vi "observacao_0MQ.vi"() -> ()   [LabVIEW 2012, in "Shared_160.lvlib"] (continued)
              tunnel: w81 -> [_ w133]
              frame False {
              }
              frame True {
                w134 = "\t"
                # "CÚPULA TRAVADA: Write LOG"
                n304 = String To Path(string="C:\\TCS\\LOG\\CUPULA\\TRAVOU.TXT" ("pathLogFocoString")) -> (path=w142:path)
                n305 = Open/Create/Replace File(file path (use dialog)=w142, error in=errorcluster {"status"=FALSE, "code"=0, "source"=""}, operation (0:open)=T7."open or create") -> (refnum out=w129:refnum<file>, error out=w127:errorcluster)  [unwired: 3 in, 1 out]
                n306 = Get Date/Time String(date format (0)=enum16{"short", "long", "abbreviated"}."short", want seconds? (F)=TRUE) -> (date string=w136:string, time string=w135:string)  [unwired: 1 in]
                n307 = Build Array(w136, w134, w135, w134, "ETIQUETA: ", w133, "\r\n") -> (w130:string[])
                n308 = call "TickTimeout.vi"() -> ("msTick"=w122:u32)  [unwired: 2 in, 2 out]
                n309 = Set File Position(refnum=w129, from (0:start)=enum16{"start", "end", "current"}."end", error in=w127) -> (refnum out=w128:refnum<file>, error out=w126:errorcluster)  [unwired: 1 in]
                n310 = global write "Global_Telescopio.vi" "CupTimeLock"(w122) -> ()
                n311 = Write to Text File(file (use dialog)=w128, text=w130, error in=w126) -> (refnum out=w139:refnum<file>, error out=w140:errorcluster)  [unwired: 1 in, 1 out]
                n312 = Close File(refnum=w139, error in=w140) -> ()  [unwired: 2 out]
              }
            }
            n313 = Or(x=w93, y=w94) -> (x .or. y?=w92:bool)
            n314 = Tick Count (ms)() -> (millisecond timer value=w87:u32)
            n315 = Add(x=w89, y=40000) -> (x+y=w86:i32)
            n316 = Greater Or Equal?(x=w87, y=w86) -> (x >= y?=w85:bool)
            n317 = shared-variable "My Computer\\Shared_160.lvlib\\Beep"(w92) -> ()  [unwired: 1 in, 1 out]
            n318 = And(x=w85, y=w84) -> (x .and. y?=w83:bool)
            n319 = case shown="True" w83 {
              frame False {
              }
              frame True {
                w203 = u16 4 items=["ZERO", "AH", "DEC", "TUBO", "CUP"] ("Controlador")
                # "Envia o comando para o\ncontrolador da cupula, após 40 segundos"
                n320 = local write "sendCommandShutter"(FALSE ("writeShutterLog")) -> ()
                n321 = call "Monta Comando.vi"("Comando"="PARAR", "Dispositivo"="TRAPEIRA" ("Comando"), "Controlador"=w203) -> ()  [unwired: 4 in, 3 out]
              }
            }
            n322 = call "Sideral_Time.vi"("Fuso"=-3.0) -> ("TU"=→"UT":string, "Sideral Time"=w110:dbl)  [unwired: 2 in, 1 out]
            n323 = global write "Global_Telescopio.vi" "Sideral Time"(w110) -> ()
          }
          frame #1 {
            w317 = u16 9 items=["Alarme", "Atencao", "Erro", "Ocupado", "Protecao", "Embreagem", "Tracking", "Var. Track", "Rápido", "Ligeiro", "Médio", "Lento", "Em movimento", ""] ("NomeStatus")
            w318 = u16 9 items=["Alarme", "Atencao", "Erro", "Ocupado", "Protecao", "Embreagem", "Tracking", "Var. Track", "Rápido", "Ligeiro", "Médio", "Lento", "Em movimento", ""] ("NomeStatus")
            w321 = u16 8 items=["Alarme", "Atencao", "Erro", "Ocupado", "Protecao", "Embreagem", "Tracking", "Var. Track", "Rápido", "Ligeiro", "Médio", "Lento", "Em movimento", ""] ("NomeStatus")
            w322 = u16 8 items=["Alarme", "Atencao", "Erro", "Ocupado", "Protecao", "Embreagem", "Tracking", "Var. Track", "Rápido", "Ligeiro", "Médio", "Lento", "Em movimento", ""] ("NomeStatus")
            w328 = 6.283185307179586
            # "Desabilita botões \"Precess\" e \"Clear\"\ndurante o apontamento"
            # "MUDANÇA:\nBit EMBREAGEM trocado pelos bits RAPIDO e LIGEIRO para detectar a retirada do objeto da posição centrada."
            # "MUDANÇA FUTURA:\nTrocar globais de calagem por valores \"latch\" dessas globais. Finalidade: manter display de coordenadas consistentes mesmo quando o usuário zerar as calagens, especialmente a local, para o próximo apontamento."
            # "ATUALIZA \nINDICADORES \nDO PAINEL"
            n324 = local read "ChkCalGlobal"() -> (w333:bool)
            n325 = global read "Global_Telescopio.vi" "PosDEC"() -> (w336:dbl)
            n326 = global read "Global_Telescopio.vi" "Sideral Time"() -> (w338:dbl)
            n327 = global read "Global_Telescopio.vi" "ObjCentrado"() -> (w310:bool)
            "ObjCentrado" <- w310
            n328 = global read "Global_Telescopio.vi" "PosAH"() -> (w337:dbl)
            n329 = call "Calcula epoch.vi"() -> ("epoch"=→"Epoch":dbl)  [unwired: 2 in]
            n330 = call "Bit Status AH.vi"("NomeStatus"=w322) -> ("StatBit"=w320:bool)
            n331 = call "Bit Status AH.vi"("NomeStatus"=w317) -> ("StatBit"=w316:bool)
            n332 = call "Bit Status DEC.vi"("NomeStatus"=w321) -> ("StatBit"=w314:bool)
            n333 = call "Bit Status DEC.vi"("NomeStatus"=w318) -> ("StatBit"=w315:bool)
            n334 = local read "LedPointing"() -> (w305:bool)
            n335 = Tick Count (ms)() -> (millisecond timer value=w306:u32)
            n336 = Compound Arithmetic op=OR(w320, w316, w314, w315) -> (w319:bool)
            n337 = case shown="True" w319 {
              frame False {
              }
              frame True {
                n338 = global write "Global_Telescopio.vi" "ObjCentrado"(FALSE) -> ()
              }
            }
            n339 = case shown="False" w305 {
              frame False {
                w344 = 0
                n340 = property on="BtPointPrecess" class="Bool"("DisabledEnum"=w344) -> ()  [unwired: 2 in, 2 out]
                n341 = property on="BtPointObjClear" class="Bool"("DisabledEnum"=w344) -> ()  [unwired: 2 in, 2 out]
              }
              frame True {
                w345 = 2
                n342 = property on="BtPointPrecess" class="Bool"("DisabledEnum"=w345) -> ()  [unwired: 2 in, 2 out]
                n343 = property on="BtPointObjClear" class="Bool"("DisabledEnum"=w345) -> ()  [unwired: 2 in, 2 out]
              }
            }
            n344 = case shown="True" w310 {
              tunnel: [w415 w432] -> w330
              tunnel: [w414 w431] -> w326
              tunnel: [w417 w435] -> w304
              tunnel: [w416 w433] -> w323
              tunnel: w338 -> [w415 w432]
              tunnel: w337 -> [w420 _]
              tunnel: w336 -> [w419 _]
              tunnel: w333 -> [w418 _]
              tunnel: [w413 w429] -> _
              tunnel: w306 -> [w413 w429]
              frame False {
                n345 = case shown="True" w418 {
                  tunnel: w419 -> [w422 w428]
                  tunnel: [w422 w427] -> w417
                  tunnel: w420 -> [w421 w426]
                  tunnel: [w421 w423] -> w416
                  frame False {
                  }
                  frame True {
                    n346 = global read "Global_Telescopio.vi" "Calagem AH"() -> (w424:dbl)
                    n347 = global read "Global_Telescopio.vi" "Calagem DEC"() -> (w425:dbl)
                    n348 = Subtract(x=w426, y=w424) -> (x-y=w423:dbl)
                    n349 = Subtract(x=w428, y=w425) -> (x-y=w427:dbl)
                  }
                }
                n350 = Subtract(x=w415, y=w416) -> (x-y=w414:dbl)
              }
              frame True {
                # "PROCESSO PRECESSÃO"
                n351 = local read "Temp amb"() -> (w438:string)
                n352 = local read "hum local"() -> (w436:string)
                n353 = local read "MeanDEC"() -> (w439:string)
                n354 = local read "pressão atm"() -> (w437:string)
                n355 = local read "PM_RA"() -> (w434:string)
                n356 = local read "MeanRA"() -> (w440:string)
                n357 = local read "PM_DEC"() -> (w430:string)
                n358 = call "PrecessFortran.vi"("Asc reta"=w440, "Var RA"=w434, "Declinação"=w439, "Temperatura (Kelvin)"=w438, "Pressao atmosferica (mB)"=w437, "Humidade relativa (0 a 1)"=w436, "Var DEC"=w430) -> ("Observed RA (radians)"=w431:dbl, "Observed Dec (radians)"=w435:dbl)  [unwired: 2 in, 5 out]
                n359 = Subtract(x=w432, y=w431) -> (x-y=w433:dbl)
              }
            }
            "AtualDEC" <- w304
            n360 = case shown="True" w310 {
              tunnel: [w366 w369] -> w335
              tunnel: [w366 w368] -> w334
              tunnel: w304 -> [_ w367]
              frame False {
                w366 = 0.0
              }
              frame True {
                n361 = stacked-sequence {
                  seq-local: [w370 _ _] -> [_ _ w408]
                  tunnel: [_ w377 _] -> w369
                  tunnel: [_ w376 _] -> w368
                  tunnel: w367 -> [_ w371 _]
                  frame #0 {
                    n362 = Tick Count (ms)() -> (millisecond timer value=w370:u32)
                  }
                  frame #1 {
                    w378 = u16 3 items=["Alarme", "Atencao", "Erro", "Ocupado", "Protecao", "Embreagem", "Tracking", "Var. Track", "Rápido", "Ligeiro", "Médio", "Lento", "Em movimento", ""] ("NomeStatus")
                    w379 = u16 3 items=["Alarme", "Atencao", "Erro", "Ocupado", "Protecao", "Embreagem", "Tracking", "Var. Track", "Rápido", "Ligeiro", "Médio", "Lento", "Em movimento", ""] ("NomeStatus")
                    # "PROCESSO LEITURA POS_MOTOR"
                    n363 = local read "MOV_IDX_AH"() -> (w374:bool)
                    n364 = local read "MOV_IDX_DEC"() -> (w372:bool)
                    n365 = call "Bit Status AH.vi"("NomeStatus"=w379) -> ("StatBit"=w375:bool)
                    n366 = call "Bit Status DEC.vi"("NomeStatus"=w378) -> ("StatBit"=w373:bool)
                    n367 = case shown="False" w375 {
                      tunnel: w371 -> [w393 _]
                      tunnel: [w392 w407] -> w377
                      tunnel: w374 -> [w391 _]
                      frame False {
                        n368 = case shown="False" w391 {
                          tunnel: w393 -> [w401 _]
                          tunnel: [w397 w406] -> w392
                          frame False {
                            w404 = u16 1 items=["ZERO", "AH", "DEC", "TUBO", "CUP"] ("Controlador")
                            # "RA"
                            # "AH"
                            n369 = call "Get Posic Motor Indexer.vi"("Controlador"=w404) -> ("PosMotor"=w395:dbl)
                            n370 = global read "Global_Telescopio.vi" "AcumPrecRA"() -> (w398:dbl)
                            n371 = Negate(x=w395) -> (-x=w396:dbl)
                            n372 = Subtract(x=w396, y=w398) -> (x-y=w405:dbl)
                            n373 = global read "Global_Telescopio.vi" "AcumAG RA"() -> (w399:dbl)
                            n374 = Cosine(x=w401) -> (cos(x)=w400:dbl)
                            n375 = Absolute Value(x=w400) -> (abs(x)=w394:dbl)
                            n376 = Subtract(x=w405, y=w399) -> (x-y=w403:dbl)
                            n377 = Multiply(x=w394, y=w403) -> (x*y=w402:dbl)
                            n378 = call "Rad to Arcsec.vi"("Radiano"=w402) -> ("Arcsec"=w397:dbl)
                          }
                          frame True {
                            n379 = local read "Offset RA"() -> (w406:dbl)
                          }
                        }
                      }
                      frame True {
                        n380 = local read "Offset RA"() -> (w407:dbl)
                      }
                    }
                    n381 = case shown="False" w373 {
                      tunnel: [w381 w390] -> w376
                      tunnel: w372 -> [w380 _]
                      frame False {
                        n382 = case shown="False" w380 {
                          tunnel: [w382 w389] -> w381
                          frame False {
                            w385 = u16 2 items=["ZERO", "AH", "DEC", "TUBO", "CUP"] ("Controlador")
                            n383 = call "Get Posic Motor Indexer.vi"("Controlador"=w385) -> ("PosMotor"=w387:dbl)
                            n384 = global read "Global_Telescopio.vi" "AcumPrecDEC"() -> (w383:dbl)
                            n385 = Subtract(x=w387, y=w383) -> (x-y=w388:dbl)
                            n386 = global read "Global_Telescopio.vi" "AcumAG DEC"() -> (w384:dbl)
                            n387 = Subtract(x=w388, y=w384) -> (x-y=w386:dbl)
                            n388 = call "Rad to Arcsec.vi"("Radiano"=w386) -> ("Arcsec"=w382:dbl)
                          }
                          frame True {
                            n389 = local read "Offset DEC"() -> (w389:dbl)
                          }
                        }
                      }
                      frame True {
                        n390 = local read "Offset DEC"() -> (w390:dbl)
                      }
                    }
                  }
                  frame #2 {
                    n391 = flat-sequence {
                      tunnel: w408 -> [w409]
                      frame #0 {
                        n392 = Tick Count (ms)() -> (millisecond timer value=w410:u32)
                        n393 = Subtract(x=w410, y=w410) -> (x-y=→"dtAUX2":u32)
                        n394 = Subtract(x=w410, y=w409) -> (x-y=→"dtAUX3":u32)
                      }
                    }
                  }
                }
              }
            }
            "Offset RA" <- w335
            "Offset DEC" <- w334
            n395 = Add(x=w328, y=w326) -> (x+y=w327:dbl)
            n396 = Add(x=w328, y=w330) -> (x+y=w331:dbl)
            n397 = Less Than 0?(x=w330) -> (x < 0?=w332:bool)
            n398 = Less Than 0?(x=w326) -> (x < 0?=w329:bool)
            n399 = call "Normliza_AH.vi"("PosAH"=w323) -> ("Numeric"=w309:dbl)
            n400 = Select(t=w331, s=w332, f=w330) -> (s? t:f=w311:dbl)
            n401 = Select(t=w327, s=w329, f=w326) -> (s? t:f=w312:dbl)
            n402 = case shown="True" w310 {
              tunnel: ["" w353] -> w313
              tunnel: w312 -> [_ w350]
              tunnel: w311 -> [_ w351]
              tunnel: w304 -> [_ w352]
              frame False {
              }
              frame True {
                n403 = disable-structure shown="Disabled" {
                  disable-tunnel: w352 -> [w364 _]
                  disable-tunnel: w351 -> [w363 _]
                  disable-tunnel: w350 -> [w362 _]
                  disable-tunnel: [w361 _] -> _
                  frame Disabled {
                    n404 = call "Hora_Limite.vi"("Asc Reta RA rad"=w362, "Sideral Time rad"=w363, "Declinação rad"=w364) -> ("TO Tempo de Observação Horas"=w361:dbl)  [unwired: 2 in]
                  }
                  frame Enabled {
                  }
                }
                n405 = call "Novo_tempo_obs.vi"() -> ("TO rad"=w348:dbl)  [unwired: 10 in, 1 out]
                n406 = Greater Than 0?(x=w348) -> (x > 0?=w347:bool)
                n407 = case shown="True" w347 {
                  tunnel: [w355 w358] -> w349
                  tunnel: w348 -> [w355 w357]
                  frame False {
                  }
                  frame True {
                    n408 = Random Number (0-1)() -> (number: 0 to 1=w359:dbl)
                    n409 = Multiply(x=w359, y=7.27e-05) -> (x*y=w356:dbl)
                    n410 = Add(x=w357, y=w356) -> (x+y=w358:dbl)
                  }
                }
                n411 = call "rad_hms.vi"("TRUE=HORA\nFALSE=GRAU"=TRUE ("TRUE=HORA\nFALSE=GRAU"), "Radiano"=w349) -> ("Hora/Graus Texto Decimal"=w353:string)  [unwired: 3 in]
              }
            }
            "Time to Limit" <- w313
            n412 = global write "Global_Telescopio.vi" "AH_now"(w309) -> ()
            n413 = call "rad_hms.vi"("TRUE=HORA\nFALSE=GRAU"=TRUE ("TRUE=HORA\nFALSE=GRAU"), "Radiano"=w311) -> ("Hora/Graus Texto Decimal"=w325:string)  [unwired: 3 in]
            "Sideral time" <- w325
            n414 = call "rad_hms.vi"("TRUE=HORA\nFALSE=GRAU"=TRUE, "Radiano"=w312) -> ("Hora/Graus Texto Decimal"=w324:string)  [unwired: 3 in]
            "Right Ascention" <- w324
            n415 = call "rad_hms.vi"("TRUE=HORA\nFALSE=GRAU"=TRUE, "Radiano"=w309) -> ("Hora/Graus Texto Decimal"=w308:string)  [unwired: 3 in]
            "Hour Angle" <- w308
            "Hour Angle 2" <- w308
            n416 = call "rad_hms.vi"("TRUE=HORA\nFALSE=GRAU"=FALSE, "Radiano"=w304) -> ("Hora/Graus Texto Decimal"=w307:string)  [unwired: 3 in]
            "Declination" <- w307
            "DEC" <- w307
            n417 = global write "Global_Telescopio.vi" "Right Ascention"(w324) -> ()
            n418 = global write "Global_Telescopio.vi" "Hour Angle"(w308) -> ()
            n419 = global write "Global_Telescopio.vi" "Sideral time"(w325) -> ()
            n420 = global write "Global_Telescopio.vi" "Declination"(w307) -> ()
            n421 = global write "Global_Telescopio.vi" "delta_now"(w304) -> ()
          }
          frame #2 {
            w464 = -0.39330025  # LatOPD rad
            # "ALTERAÇÃO FEITA EM 12/12/2012\nFEITA PARA RESOLVER EXCESSÍVOS\nMOVIMENTOS DO ACOMP.SID. DA\nCÚPULA (DANIEL). A condição de statCUP=0 foi inserida em 08/5/2013-> Só corrige a cúpula se esta estiver parada!"
            # "Horas"
            # "MUDANÇA FUTURA:\nPassar LatOPD para Global"
            # "az"
            # "z"
            # "Cálculo do Azimute da Cúpula e Hab Acompanham. Cúpula"
            # "Lógica de Segurança"
            # "ANGULO ZENITAL"
            n422 = global read "Global_Telescopio.vi" "OffsetCupula"() -> (w473:dbl)
            n423 = global read "Global_Telescopio.vi" "AH_now"() -> (w456:dbl)
            n424 = global read "Global_Telescopio.vi" "delta_now"() -> (w463:dbl)
            n425 = global read "Global_Telescopio.vi" "Limite EAST"() -> (w457:dbl)
            n426 = global read "Global_Telescopio.vi" "Limite WEST"() -> (w458:dbl)
            n427 = call "Calculo_do_Azimute_da_Cupula_2.vi"("AH"=w456, "DEC"=w463, "OffsetTCSPD"=w473) -> ("PosCup"=w442:u16)  [unwired: 3 in, 1 out]
            "Azimute cup" <- w442
            n428 = local read "Tick Cupula"() -> (w448:u32)
            n429 = Tick Count (ms)() -> (millisecond timer value=w449:u32)
            n430 = global read "Global_Telescopio.vi" "PosCUP"() -> (→"PosCUP":i16)
            n431 = Multiply(x=w456, y=3.8197) -> (x*y=w459:dbl)
            n432 = call "Altura_e_Azimute.vi"("LAT rad"=w464, "DEC rad"=w463, "AH rad"=w456) -> ("AZIMUTE graus"=w444:dbl, "ANG. ZENITAL graus"=w462:dbl, "AZIMUTE rad"=w465:dbl, "ANG. ZENITAL rad"=w466:dbl)  [unwired: 2 out]
            "Azimuth" <- w444
            "Zenital angle" <- w462
            n433 = Greater Or Equal?(x=w449, y=w448) -> (x >= y?=w447:bool)
            n434 = Greater?(x=w459, y=w457) -> (0:w455:bool)
            n435 = Less?(x=w459, y=w458) -> (x < y?=w454:bool)
            n436 = call "Checa destino cupula.vi"("Target"=w442) -> ("moverCup"=w441:bool)  [unwired: 6 in, 2 out]
            n437 = local read "statCUP"() -> (w446:i32)
            n438 = Not And(1:w454, 2:w455) -> (0:w451:bool)
            n439 = Equal To 0?(x=w446) -> (x = 0?=w445:bool)
            n440 = call "Calcula_Proteção.vi"("Zenital angle rad"=w466, "Azimute rad"=w465) -> ("Z_SEGURANÇA_GRAUS"=w475:dbl, "Prot Segur"=w477:bool, "Z_LIBERA_GRAUS"=w474:dbl, "Z_MAX_GRAUS"=w476:dbl, "Prot Zmax"=w452:bool)
            n441 = Compound Arithmetic op=AND(w441, "DOME", w447, w445) -> (w472:bool)
            n442 = case shown="True" w472 {
              tunnel: w442 -> [_ w481]
              tunnel: FALSE -> [_ w486]
              frame False {
              }
              frame True {
                # "TEMPO CÚPULA"
                # "2m Tempo para novo movimento"
                n443 = Tick Count (ms)() -> (millisecond timer value=w485:u32)
                n444 = local write "Dome on Target"(w486) -> ()
                n445 = To Word Integer(number=w481) -> (16bit integer=w482:i16)
                n446 = Add(x=w485, y=u32 120000) -> (x+y=→"Tick Cupula":u32)
                n447 = local write "statCUP"(1 ("statCUP")) -> ()
                n448 = Number To Decimal String(number=w481) -> (decimal integer string=→"TargetCup":string)  [unwired: 1 in]
                n449 = global write "Global_Telescopio.vi" "TargetCUP"(w482) -> ()
              }
            }
            n450 = global write "Global_Telescopio.vi" "Z_SEGURANÇA_GRAUS"(w475) -> ()
            n451 = global write "Global_Telescopio.vi" "Zenital angle GRAUS"(w462) -> ()
            n452 = global write "Global_Telescopio.vi" "Azimute GRAUS"(w444) -> ()
            n453 = global write "Global_Telescopio.vi" "Z_MAX_GRAUS"(w476) -> ()
            n454 = global write "Global_Telescopio.vi" "Z_LIBERA_GRAUS"(w474) -> ()
            n455 = global read "Global_Telescopio.vi" "LIMITE"() -> (w471:bool)
            n456 = Or(x=w451, y=w452) -> (x .or. y?=w453:bool)
            n457 = Or(x=w471, y=w453) -> (x .or. y?=w470:bool)
            "Proteção" <- w470
            n458 = call "Borda_Subida_Z_max.vi"("Entrada"=w470) -> ("Boolean"=w479:bool)
            n459 = call "Borda_Subida_Segurança.vi"("Entrada"=w477) -> ("Boolean"=w478:bool)
            n460 = case shown="True" w479 {
              frame False {
              }
              frame True {
                w494 = FALSE
                w492 = "Telescópio parado por inclinação excessiva!" ("SYSTEM MESSAGES")
                n461 = local write "LED MOUNT"(w494) -> ()
                n462 = local write "MOUNT"(w494) -> ()
                n463 = global write "Global_Telescopio.vi" "ObjCentrado"(FALSE) -> ()
                n464 = global write "Global_Telescopio.vi" "STOP ALL"(TRUE ("STOP ALL")) -> ()
                n465 = call "Monta_Mensagem.vi"("Mensagem"=w492) -> ()  [unwired: 2 in]
                n466 = call "Salva_systems_messages.vi"("Mensagem"=w492) -> ()  [unwired: 5 in]
              }
            }
            n467 = Select(t=u8 2 ("Disabled"), s=w470, f=u8 0 ("Disabled")) -> (s? t:f=w467:u8)
            n468 = case shown="True" w478 {
              frame False {
              }
              frame True {
                w490 = u16 2 items=["ZERO", "AH", "DEC", "TUBO", "CUP"] ("Controlador")
                w489 = "FREAR" ("Comando")
                w491 = u16 1 items=["ZERO", "AH", "DEC", "TUBO", "CUP"] ("Controlador")
                w488 = "EIXO" ("Dispositivo")
                n469 = call "Monta Comando.vi"("Comando"=w489, "Dispositivo"=w488, "Controlador"=w491) -> ()  [unwired: 4 in, 3 out]
                n470 = call "Monta Comando.vi"("Comando"=w489, "Dispositivo"=w488, "Controlador"=w490) -> ()  [unwired: 4 in, 3 out]
              }
            }
            n471 = property on="MOUNT" class="Bool (strict)"("Disabled"=w467) -> ()  [unwired: 2 in, 2 out]
            "Led Chave Dome" <- "DOME"
          }
          frame #3 {
            w501 = u32 500 ("millisecond multiple")
            w515 = u16 3 items=["Alarme", "Atencao", "Erro", "Ocupado", "TBD", "LCB", "Trapeira", "Paravento", "DomoRap", "DomoCW", "DomoCCW", "TBD", "Em movimento", "TBD"] ("NomeStatus")
            w527 = u16 3 items=["Alarme", "Atencao", "Erro", "Ocupado", "Protecao", "Embreagem", "Tracking", "Var. Track", "Rápido", "Ligeiro", "Médio", "Lento", "Em movimento", ""] ("NomeStatus")
            w528 = u16 3 items=["Alarme", "Atencao", "Erro", "Ocupado", "Protecao", "Embreagem", "Tracking", "Var. Track", "Rápido", "Ligeiro", "Médio", "Lento", "Em movimento", ""] ("NomeStatus")
            # "04-07-2022\nValor de Erro PROTEC\nalterado de 5 para 10"
            # "MUDANÇA: \nIncluído CASE"
            # "Esse metrônomo determina\no ciclo de 0,5 segundo dos\ncálculos rápidos e totais!"
            # "PROCESSO APONTAMENTO"
            # "MÁQUINA DE ESTADO DO APONTAMENTO"
            # "Seta nome para GO/STOP"
            n472 = global read "Global_Telescopio.vi" "PosDEC"() -> (w530:dbl)
            n473 = global read "Global_Telescopio.vi" "TargetDEC"() -> (w531:dbl)
            n474 = global read "Global_Telescopio.vi" "LimiarRapMed"() -> (w529:dbl)
            n475 = global read "Global_Telescopio.vi" "ErroMaxEixo"() -> (w518:dbl)
            n476 = call "Bit Status DEC.vi"("NomeStatus"=w527) -> ("StatBit"=w517:bool)
            n477 = global read "Global_Telescopio.vi" "Sideral Time"() -> (w509:dbl)
            n478 = global read "Global_Telescopio.vi" "PosAH"() -> (w532:dbl)
            n479 = global read "Global_Telescopio.vi" "TargetRA"() -> (w533:dbl)
            n480 = global write "Global_Telescopio.vi" "Estado AH"("statAH") -> ()
            n481 = call "Bit Status AH.vi"("NomeStatus"=w528) -> ("StatBit"=w516:bool)
            n482 = global write "Global_Telescopio.vi" "Estado DEC"("statDEC") -> ()
            n483 = case shown="1" "statDEC" {
              selector: "statDEC" -> [w663 _ _ _ _ _ _ _ _]
              tunnel: [w663 w670 w700 w722 w749 w773 0 ("t") w790 w795] -> w510
              tunnel: w531 -> [_ w669 _ w716 _ _ _ _ _]
              tunnel: w530 -> [_ w665 _ w719 _ _ _ _ _]
              tunnel: w518 -> [_ _ _ w720 _ _ _ _ _]
              tunnel: w529 -> [_ w671 _ _ _ _ _ _ _]
              tunnel: w517 -> [_ w668 _ w715 _ _ _ _ _]
              frame 0, Default {
                w661 = 0 ("CR DEC")
                # "Sem apontamento"
                n484 = call "TickTimeout.vi"() -> ("msTick"=→"TimeoutDEC":u32)  [unwired: 2 in, 2 out]
                n485 = local write "CR DEC"(w661) -> ()
                n486 = local write "C. DEC"(w661) -> ()
              }
              frame 1 {
                # "Envia\nComando"
                n487 = Subtract(x=w669, y=w665) -> (x-y=w667:dbl)
                n488 = Absolute Value(x=w667) -> (abs(x)=w672:dbl)
                n489 = local write "dec="(FALSE ("dec=")) -> ()
                n490 = Less?(x=w672, y=w671) -> (x < y?=w666:bool)
                n491 = case shown="False" w666 {
                  tunnel: [w676 3] -> w670
                  tunnel: w669 -> [w675 _]
                  tunnel: w667 -> [w674 _]
                  tunnel: w668 -> [w673 _]
                  frame False {
                    # "destino"
                    # "Fora do"
                    n492 = case shown="False" w673 {
                      tunnel: [w680 w688] -> w676
                      tunnel: w675 -> [w683 _]
                      tunnel: w674 -> [_ _]
                      frame False {
                        w687 = u16 2 items=["ZERO", "AH", "DEC", "TUBO", "CUP"] ("Controlador")
                        # "limpa flag"
                        # "CLP Pronto"
                        n493 = local write "Flag ativo DEC"(FALSE ("Flag ativo DEC")) -> ()
                        n494 = call "rad_hms.vi"("TRUE=HORA\nFALSE=GRAU"=FALSE, "Radiano"=w683) -> ("Hora/Graus Texto Decimal"=w684:string)  [unwired: 3 in]
                        n495 = call "Monta Comando.vi"("Set Point"=w684, "Comando"="MOVER_RAP", "Dispositivo"="EIXO" ("Comando"), "Controlador"=w687) -> ("Erro Comunicação"=w678:bool)  [unwired: 3 in, 2 out]
                        n496 = Select(t=6, s=w678, f=20) -> (s? t:f=w680:i32)
                      }
                      frame True {
                        # "CLP Ocupado"
                        n497 = local read "TimeoutDEC"() -> (w690:u32)
                        n498 = call "TickTimeout.vi"("msInicial"=w690, "msTimeout"=u32 4000) -> ("Timeout"=w689:bool)  [unwired: 2 out]
                        n499 = case shown="False" w689 {
                          tunnel: [1 5] -> w688
                          frame False {
                          }
                          frame True {
                            # "Tratar\nTimeout"
                          }
                        }
                      }
                    }
                  }
                  frame True {
                    # "Dist. pequena p/ mov. rápido"
                    # "Ligar mov. lento"
                    n500 = call "TickTimeout.vi"() -> ("msTick"=w694:u32)  [unwired: 2 in, 2 out]
                    n501 = local write "TimeoutDEC"(w694) -> ()
                  }
                }
              }
              frame 2 {
                w701 = u16 12 items=["Alarme", "Atencao", "Erro", "Ocupado", "Protecao", "Embreagem", "Tracking", "Var. Track", "Rápido", "Ligeiro", "Médio", "Lento", "Em movimento", ""] ("NomeStatus")
                # "Aguarda fim mov. Rap."
                n502 = global read "Global_Telescopio.vi" "Habilita supervisao"() -> (w697:bool)
                n503 = call "Bit Status DEC.vi"("NomeStatus"=w701) -> ("StatBit"=w702:bool)
                n504 = case shown="True" w702 {
                  tunnel: [1 w711] -> w699
                  frame False {
                    # "Motor parado.\nTestar se chegou\nao destino"
                    n505 = call "TickTimeout.vi"() -> ("msTick"=w707:u32)  [unwired: 2 in, 2 out]
                    n506 = local write "TimeoutDEC"(w707) -> ()
                  }
                  frame True {
                    # "Ainda movendo...\nAGUARDAR"
                    n507 = local read "Erro PROTEC"() -> (w713:i32)
                    n508 = call "PROTECAO_DEC.vi"() -> ("CONT DEC"=w714:i32)  [unwired: 11 in]
                    "C. DEC" <- w714
                    n509 = Greater Or Equal?(x=w714, y=w713) -> (x >= y?=w709:bool)
                    n510 = Select(t=6, s=w709, f=2) -> (s? t:f=w711:i32)
                  }
                }
                n511 = case shown="True" w697 {
                  tunnel: [FALSE w706] -> w696
                  frame False {
                  }
                  frame True {
                    n512 = local read "Erro Lim"() -> (w704:i32)
                    n513 = Greater Or Equal?(x="CR DEC", y=w704) -> (x >= y?=w706:bool)
                  }
                }
                n514 = Select(t=6, s=w696, f=w699) -> (s? t:f=w700:i32)
              }
              frame 3 {
                # "Mov.Lento"
                n515 = Subtract(x=w716, y=w719) -> (x-y=w717:dbl)
                n516 = Absolute Value(x=w717) -> (abs(x)=w721:dbl)
                n517 = Less Or Equal?(x=w721, y=w720) -> (x <= y?=w718:bool)
                n518 = case shown="False" w718 {
                  selector: w718 -> [_ w745]
                  tunnel: [w724 0] -> w722
                  tunnel: w717 -> [w723 _]
                  tunnel: w716 -> [_ w744]
                  tunnel: w715 -> [w725 _]
                  frame False {
                    n519 = case shown="False" w725 {
                      tunnel: [w729 w738] -> w724
                      tunnel: w723 -> [w732 _]
                      frame False {
                        w737 = u16 2 items=["ZERO", "AH", "DEC", "TUBO", "CUP"] ("Controlador")
                        # "limpa flag"
                        # "Mov. lento"
                        n520 = call "rad_hms.vi"("TRUE=HORA\nFALSE=GRAU"=FALSE ("TRUE=HORA\nFALSE=GRAU"), "Radiano"=w732) -> ("Hora/Graus Texto Decimal"=w734:string)  [unwired: 3 in]
                        n521 = call "Monta Comando.vi"("Set Point"=w734, "Comando"="MOVER_REL", "Dispositivo"="EIXO" ("Comando"), "Controlador"=w737) -> ("Erro Comunicação"=w727:bool)  [unwired: 3 in, 2 out]
                        n522 = call "TickTimeout.vi"() -> ("msTick"=w731:u32)  [unwired: 2 in, 2 out]
                        n523 = local write "Flag ativo DEC"(FALSE ("Flag ativo DEC")) -> ()
                        n524 = local write "TimeoutDEC"(w731) -> ()
                        n525 = Select(t=6, s=w727, f=40) -> (s? t:f=w729:i32)
                      }
                      frame True {
                        # "CLP Ocupado"
                        n526 = local read "TimeoutDEC"() -> (w740:u32)
                        n527 = call "TickTimeout.vi"("msInicial"=w740, "msTimeout"=u32 2000) -> ("Timeout"=w739:bool)  [unwired: 2 out]
                        n528 = case shown="False" w739 {
                          tunnel: [3 5] -> w738
                          frame False {
                          }
                          frame True {
                          }
                        }
                      }
                    }
                  }
                  frame True {
                    # "DEC no destino"
                    n529 = local write "LatchDeslocDEC"(w744) -> ()
                    "DEC on Target" <- w745
                  }
                }
              }
              frame 4 {
                w752 = u16 12 items=["Alarme", "Atencao", "Erro", "Ocupado", "Protecao", "Embreagem", "Tracking", "Var. Track", "Rápido", "Ligeiro", "Médio", "Lento", "Em movimento", ""] ("NomeStatus")
                # "Aguarda fim mov. lento"
                n530 = global read "Global_Telescopio.vi" "Habilita supervisao"() -> (w750:bool)
                n531 = call "Bit Status DEC.vi"("NomeStatus"=w752) -> ("StatBit"=w753:bool)
                n532 = case shown="True" w753 {
                  tunnel: [3 w763] -> w748
                  frame False {
                    # "Motor parado.\nTestar se chegou\nao destino"
                    n533 = call "TickTimeout.vi"() -> ("msTick"=w758:u32)  [unwired: 2 in, 2 out]
                    n534 = local write "TimeoutDEC"(w758) -> ()
                  }
                  frame True {
                    n535 = local read "Erro PROTEC"() -> (w765:i32)
                    n536 = call "PROTECAO_DEC.vi"() -> ("CONT DEC"=w760:i32)  [unwired: 11 in]
                    n537 = local write "C. DEC"(w760) -> ()
                    n538 = Greater Or Equal?(x=w760, y=w765) -> (x >= y?=w762:bool)
                    n539 = local read "TimeoutDEC"() -> (w767:u32)
                    n540 = call "TickTimeout.vi"("msInicial"=w767, "msTimeout"=u32 4000) -> ("Timeout"=w766:bool)  [unwired: 2 out]
                    n541 = case shown="False" w766 {
                      tunnel: [4 5] -> w761
                      frame False {
                      }
                      frame True {
                      }
                    }
                    n542 = Select(t=6, s=w762, f=w761) -> (s? t:f=w763:i32)
                  }
                }
                n543 = case shown="True" w750 {
                  tunnel: [FALSE w757] -> w747
                  frame False {
                  }
                  frame True {
                    n544 = local read "CR DEC"() -> (w756:i32)
                    n545 = local read "Erro Lim"() -> (w755:i32)
                    n546 = Greater Or Equal?(x=w756, y=w755) -> (x >= y?=w757:bool)
                  }
                }
                n547 = Select(t=6, s=w747, f=w748) -> (s? t:f=w749:i32)
              }
              frame 5 {
                w778 = u16 2 items=["ZERO", "AH", "DEC", "TUBO", "CUP"] ("Controlador")
                # "Reiniciar apontamento"
                # "Trata Timeout"
                n548 = call "TickTimeout.vi"() -> ("msTick"=w775:u32)  [unwired: 2 in, 2 out]
                n549 = local write "TimeoutDEC"(w775) -> ()
                n550 = call "Monta Comando.vi"("Comando"="PARAR", "Dispositivo"="PROG" ("Comando"), "Controlador"=w778) -> ("Erro Comunicação"=w771:bool)  [unwired: 4 in, 2 out]
                n551 = Select(t=6, s=w771, f=1) -> (s? t:f=w773:i32)
              }
              frame 6 {
                # "PARADA POR ERRO DO CONTROLADOR"
                n552 = stacked-sequence {
                  frame #0 {
                    w781 = u16 2 items=["ZERO", "AH", "DEC", "TUBO", "CUP"] ("Controlador")
                    n553 = call "Monta Comando.vi"("Comando"="PARAR", "Dispositivo"="PROG" ("Comando"), "Controlador"=w781) -> ()  [unwired: 4 in, 3 out]
                    "dec=" <- TRUE ("ah=")
                  }
                  frame #1 {
                    w784 = "Erro de Controlador DEC , REAPONTAR !" ("Mensagem")
                    n554 = local write "Flag de erro p/ apagar lampada"(TRUE ("Flag de erro p/ apagar lampada")) -> ()
                    n555 = call "Monta_Mensagem.vi"("Mensagem"=w784) -> ()  [unwired: 2 in]
                    n556 = call "Salva_systems_messages.vi"("Mensagem"=w784) -> ()  [unwired: 5 in]
                  }
                  frame #2 {
                    w787 = u16 2 items=["ZERO", "AH", "DEC", "TUBO", "CUP"] ("Controlador")
                    # "Em movimento não aceita reset"
                    # "Segundo PARAR por garantia"
                    n557 = call "Monta Comando.vi"("Comando"="PARAR", "Dispositivo"="PROG", "Controlador"=w787) -> ()  [unwired: 4 in, 3 out]
                  }
                }
              }
              frame 20 {
                # "Espera entrar\nem movimento"
                n558 = local read "Flag ativo DEC"() -> (w789:bool)
                n559 = case shown="True" w789 {
                  tunnel: [20 ("t") 2 ("t")] -> w790
                  frame False {
                  }
                  frame True {
                    # "limpa flag"
                    n560 = local write "Flag ativo DEC"(FALSE ("Flag ativo AH")) -> ()
                  }
                }
              }
              frame 40 {
                # "Espera entrar\nem movimento"
                n561 = local read "Flag ativo DEC"() -> (w794:bool)
                n562 = case shown="True" w794 {
                  tunnel: [40 ("t") 4 ("t")] -> w795
                  frame False {
                  }
                  frame True {
                    # "limpa flag"
                    n563 = local write "Flag ativo DEC"(FALSE ("Flag ativo AH")) -> ()
                  }
                }
              }
            }
            n564 = case shown="5" "statAH" {
              selector: "statAH" -> [w801 _ _ _ _ _ _ _ _ _]
              tunnel: [w801 w810 w838 w854 w878 w906 w931 0 ("t") w947 w952] -> w514
              tunnel: w509 -> [_ w807 _ _ w875 _ _ _ _ _]
              tunnel: w533 -> [_ w806 _ _ w872 _ _ _ _ _]
              tunnel: w532 -> [_ w804 _ _ w874 _ _ _ _ _]
              tunnel: w518 -> [_ _ _ _ w879 _ _ _ _ _]
              tunnel: w529 -> [_ w811 _ _ _ _ _ _ _ _]
              tunnel: w516 -> [_ w808 _ w855 w876 _ _ _ _ _]
              frame 0, Default {
                w799 = 0 ("CR AH")
                # "Sem apontamento"
                n565 = call "TickTimeout.vi"() -> ("msTick"=→"TimeoutAH":u32)  [unwired: 2 in, 2 out]
                n566 = local write "CR AH"(w799) -> ()
                n567 = local write "C. AH"(w799) -> ()
              }
              frame 1 {
                # "Mov.Rapido"
                n568 = call "Calculo_AH.vi"("AH_Telescopio"=w804, "RA_Destino"=w806, "Hora Sideral"=w807) -> ("Dif_Abs_AH"=w805:dbl, "AH_Destino"=w802:dbl)  [unwired: 1 out]
                "AH_Destino" <- w802
                n569 = Less?(x=w805, y=w811) -> (x < y?=w809:bool)
                n570 = case shown="False" w809 {
                  tunnel: w802 -> [w812 _]
                  tunnel: [w813 3] -> w810
                  tunnel: w808 -> [w814 _]
                  frame False {
                    n571 = case shown="True" w814 {
                      tunnel: w812 -> [w820 _]
                      tunnel: [w817 w826] -> w813
                      frame False {
                        w822 = u16 1 items=["ZERO", "AH", "DEC", "TUBO", "CUP"] ("Controlador")
                        # "limpa flag"
                        # "Aguardar\nfim mov."
                        # "Mov. rápido"
                        n572 = local write "Flag ativo AH"(FALSE ("Flag ativo AH")) -> ()
                        n573 = call "rad_hms.vi"("TRUE=HORA\nFALSE=GRAU"=TRUE ("TRUE=HORA\nFALSE=GRAU"), "Radiano"=w820) -> ("Hora/Graus Texto Decimal"=w825:string)  [unwired: 3 in]
                        n574 = call "Monta Comando.vi"("Set Point"=w825, "Comando"="MOVER_RAP", "Dispositivo"="EIXO" ("Comando"), "Controlador"=w822) -> ("Erro Comunicação"=w819:bool)  [unwired: 3 in, 2 out]
                        n575 = Select(t=7, s=w819, f=20) -> (s? t:f=w817:i32)
                      }
                      frame True {
                        # "CLP Ocupado"
                        n576 = local read "TimeoutAH"() -> (w828:u32)
                        n577 = call "TickTimeout.vi"("msInicial"=w828, "msTimeout"=u32 8000) -> ("Timeout"=w827:bool)  [unwired: 2 out]
                        n578 = case shown="True" w827 {
                          tunnel: [1 6] -> w826
                          frame False {
                          }
                          frame True {
                            # "Tratar\nTimeout"
                          }
                        }
                      }
                    }
                  }
                  frame True {
                    # "Ligar acomp. sideral"
                    # "Dist. pequena p/ mov. rápido"
                    n579 = call "TickTimeout.vi"() -> ("msTick"=w832:u32)  [unwired: 2 in, 2 out]
                    n580 = local write "TimeoutAH"(w832) -> ()
                  }
                }
                n581 = local write "ah="(FALSE ("ah=")) -> ()
              }
              frame 2 {
                w840 = u16 12 items=["Alarme", "Atencao", "Erro", "Ocupado", "Protecao", "Embreagem", "Tracking", "Var. Track", "Rápido", "Ligeiro", "Médio", "Lento", "Em movimento", ""] ("NomeStatus")
                # "Aguarda fim mov. Rap."
                n582 = call "Bit Status AH.vi"("NomeStatus"=w840) -> ("StatBit"=w839:bool)
                n583 = case shown="True" w839 {
                  tunnel: [1 w849] -> w837
                  frame False {
                    # "Motor parado.\nTestar se precisa\nde novo cmd. \nde mov. rápido"
                    n584 = call "TickTimeout.vi"() -> ("msTick"=w845:u32)  [unwired: 2 in, 2 out]
                    n585 = local write "TimeoutAH"(w845) -> ()
                  }
                  frame True {
                    # "Aqui também \ncaberia um \nTimeout?"
                    # "Ainda movendo...\nAGUARDAR"
                    n586 = local read "AH_Destino"() -> (w847:dbl)
                    n587 = local read "Erro PROTEC"() -> (w853:i32)
                    n588 = call "PROTECAO_AH.vi"("AH_Destino"=w847) -> ("CONT AH"=w848:i32)  [unwired: 10 in]
                    "C. AH" <- w848
                    n589 = Greater Or Equal?(x=w848, y=w853) -> (x >= y?=w852:bool)
                    n590 = Select(t=7, s=w852, f=2) -> (s? t:f=w849:i32)
                  }
                }
                n591 = global read "Global_Telescopio.vi" "Habilita supervisao"() -> (w835:bool)
                n592 = case shown="True" w835 {
                  tunnel: [FALSE w843] -> w834
                  frame False {
                  }
                  frame True {
                    n593 = local read "Erro Lim"() -> (w842:i32)
                    n594 = Greater Or Equal?(x="CR AH", y=w842) -> (x >= y?=w843:bool)
                  }
                }
                n595 = Select(t=7, s=w834, f=w837) -> (s? t:f=w838:i32)
              }
              frame 3 {
                # "Liga Acomp. Sideral"
                n596 = case shown="True" w855 {
                  tunnel: [w856 w865] -> w854
                  frame False {
                    w860 = TRUE
                    w862 = u16 1 items=["ZERO", "AH", "DEC", "TUBO", "CUP"] ("Controlador")
                    # "Usar mov. lento"
                    # "CLP Pronto - Liga sideral"
                    n597 = call "Monta Comando.vi"("Comando"="LIGAR", "Dispositivo"="SIDERAL" ("Comando"), "Controlador"=w862) -> ("Erro Comunicação"=w858:bool)  [unwired: 4 in, 2 out]
                    n598 = Select(t=7, s=w858, f=4) -> (s? t:f=w856:i32)
                    n599 = call "TickTimeout.vi"() -> ("msTick"=w861:u32)  [unwired: 2 in, 2 out]
                    n600 = local write "LED MOUNT"(w860) -> ()
                    n601 = local write "MOUNT"(w860) -> ()
                    n602 = local write "TimeoutAH"(w861) -> ()
                  }
                  frame True {
                    # "CLP Ocupado"
                    n603 = local read "TimeoutAH"() -> (w867:u32)
                    n604 = call "TickTimeout.vi"("msInicial"=w867, "msTimeout"=u32 8000) -> ("Timeout"=w866:bool)  [unwired: 2 out]
                    n605 = case shown="True" w866 {
                      tunnel: [3 6] -> w865
                      frame False {
                      }
                      frame True {
                        # "Tratar\nTimeout"
                      }
                    }
                  }
                }
              }
              frame 4 {
                # "Mov.Lento"
                n606 = call "Calculo_AH.vi"("AH_Telescopio"=w874, "RA_Destino"=w872, "Hora Sideral"=w875) -> ("Dif_AH"=w871:dbl, "Dif_Abs_AH"=w873:dbl)  [unwired: 1 out]
                n607 = Less?(x=w873, y=w879) -> (x < y?=w877:bool)
                n608 = case shown="True" w877 {
                  selector: w877 -> [_ w902]
                  tunnel: [w881 0] -> w878
                  tunnel: w876 -> [w882 _]
                  tunnel: w872 -> [_ w901]
                  tunnel: w871 -> [w880 _]
                  frame False {
                    n609 = case shown="True" w882 {
                      tunnel: [w885 w895] -> w881
                      tunnel: w880 -> [w889 _]
                      frame False {
                        w891 = u16 1 items=["ZERO", "AH", "DEC", "TUBO", "CUP"] ("Controlador")
                        # "limpa flag"
                        # "Envia Cmd. Mov. Lento"
                        n610 = call "TickTimeout.vi"() -> ("msTick"=w888:u32)  [unwired: 2 in, 2 out]
                        n611 = local write "TimeoutAH"(w888) -> ()
                        n612 = local write "Flag ativo AH"(FALSE ("Flag ativo AH")) -> ()
                        n613 = call "rad_hms.vi"("TRUE=HORA\nFALSE=GRAU"=TRUE ("TRUE=HORA\nFALSE=GRAU"), "Radiano"=w889) -> ("Hora/Graus Texto Decimal"=w894:string)  [unwired: 3 in]
                        n614 = call "Monta Comando.vi"("Set Point"=w894, "Comando"="MOVER_REL", "Dispositivo"="EIXO" ("Comando"), "Controlador"=w891) -> ("Erro Comunicação"=w884:bool)  [unwired: 3 in, 2 out]
                        n615 = Select(t=7, s=w884, f=50) -> (s? t:f=w885:i32)
                      }
                      frame True {
                        # "CLP Ocupado"
                        n616 = local read "TimeoutAH"() -> (w897:u32)
                        n617 = call "TickTimeout.vi"("msInicial"=w897, "msTimeout"=u32 8000) -> ("Timeout"=w896:bool)  [unwired: 2 out]
                        n618 = case shown="False" w896 {
                          tunnel: [4 6] -> w895
                          frame False {
                          }
                          frame True {
                          }
                        }
                      }
                    }
                  }
                  frame True {
                    # "AH on Target"
                    n619 = local write "LatchDeslocRA"(w901) -> ()
                    "RA on Target" <- w902
                  }
                }
              }
              frame 5 {
                w910 = u16 12 items=["Alarme", "Atencao", "Erro", "Ocupado", "Protecao", "Embreagem", "Tracking", "Var. Track", "Rápido", "Ligeiro", "Médio", "Lento", "Em movimento", ""] ("NomeStatus")
                # "Aguarda fim mov. Lento"
                n620 = call "Bit Status AH.vi"("NomeStatus"=w910) -> ("StatBit"=w909:bool)
                n621 = case shown="True" w909 {
                  tunnel: [4 w922] -> w904
                  frame False {
                    # "Motor parado.\nTestar se chegou\nao destino"
                    n622 = call "TickTimeout.vi"() -> ("msTick"=w915:u32)  [unwired: 2 in, 2 out]
                    n623 = local write "TimeoutAH"(w915) -> ()
                  }
                  frame True {
                    # "Trata Timeout"
                    n624 = local read "AH_Destino"() -> (w917:dbl)
                    n625 = local read "Erro PROTEC"() -> (w920:i32)
                    n626 = call "PROTECAO_AH.vi"("AH_Destino"=w917) -> ("CONT AH"=w918:i32)  [unwired: 10 in]
                    n627 = local read "TimeoutAH"() -> (w925:u32)
                    n628 = Greater Or Equal?(x=w918, y=w920) -> (x >= y?=w919:bool)
                    n629 = local write "C. AH"(w918) -> ()
                    n630 = call "TickTimeout.vi"("msInicial"=w925, "msTimeout"=u32 8000) -> ("Timeout"=w924:bool)  [unwired: 2 out]
                    n631 = case shown="False" w924 {
                      tunnel: [5 6] -> w921
                      frame False {
                      }
                      frame True {
                        # "Tratar\nTimeout"
                      }
                    }
                    n632 = Select(t=7, s=w919, f=w921) -> (s? t:f=w922:i32)
                  }
                }
                n633 = global read "Global_Telescopio.vi" "Habilita supervisao"() -> (w908:bool)
                n634 = case shown="True" w908 {
                  tunnel: [FALSE w914] -> w905
                  frame False {
                  }
                  frame True {
                    n635 = local read "Erro Lim"() -> (w912:i32)
                    n636 = local read "CR AH"() -> (w913:i32)
                    n637 = Greater Or Equal?(x=w913, y=w912) -> (x >= y?=w914:bool)
                  }
                }
                n638 = Select(t=7, s=w905, f=w904) -> (s? t:f=w906:i32)
              }
              frame 6 {
                w934 = u16 1 items=["ZERO", "AH", "DEC", "TUBO", "CUP"] ("Controlador")
                # "Reiniciar apontamento"
                # "Trata Timeout"
                n639 = call "TickTimeout.vi"() -> ("msTick"=w933:u32)  [unwired: 2 in, 2 out]
                n640 = call "Monta Comando.vi"("Comando"="PARAR", "Dispositivo"="PROG" ("Comando"), "Controlador"=w934) -> ("Erro Comunicação"=w929:bool)  [unwired: 4 in, 2 out]
                n641 = local write "TimeoutAH"(w933) -> ()
                n642 = Select(t=7, s=w929, f=1) -> (s? t:f=w931:i32)
              }
              frame 7 {
                # "PARADA POR ERRO DO CONTROLADOR"
                n643 = stacked-sequence {
                  frame #0 {
                    w939 = u16 1 items=["ZERO", "AH", "DEC", "TUBO", "CUP"] ("Controlador")
                    n644 = call "Monta Comando.vi"("Comando"="PARAR", "Dispositivo"="PROG" ("Comando"), "Controlador"=w939) -> ()  [unwired: 4 in, 3 out]
                    "ah=" <- TRUE ("ah=")
                  }
                  frame #1 {
                    w942 = "Erro de Controlador RA , REAPONTAR !" ("Mensagem")
                    n645 = call "Monta_Mensagem.vi"("Mensagem"=w942) -> ()  [unwired: 2 in]
                    n646 = call "Salva_systems_messages.vi"("Mensagem"=w942) -> ()  [unwired: 5 in]
                    "Flag de erro p/ apagar lampada" <- TRUE ("Flag de erro p/ apagar lampada")
                  }
                  frame #2 {
                    w946 = u16 1 items=["ZERO", "AH", "DEC", "TUBO", "CUP"] ("Controlador")
                    # "Em movimento não aceita reset"
                    # "Segundo PARAR por garantia"
                    n647 = call "Monta Comando.vi"("Comando"="PARAR", "Dispositivo"="PROG", "Controlador"=w946) -> ()  [unwired: 4 in, 3 out]
                  }
                }
              }
              frame 20 {
                # "Espera entrar\nem movimento"
                n648 = local read "Flag ativo AH"() -> (w948:bool)
                n649 = case shown="True" w948 {
                  tunnel: [20 ("t") 2 ("t")] -> w947
                  frame False {
                  }
                  frame True {
                    # "limpa flag"
                    n650 = local write "Flag ativo AH"(FALSE ("Flag ativo AH")) -> ()
                  }
                }
              }
              frame 50 {
                # "Espera entrar\nem movimento"
                n651 = local read "Flag ativo AH"() -> (w953:bool)
                n652 = case shown="True" w953 {
                  tunnel: [50 ("t") 5 ("t")] -> w952
                  frame False {
                  }
                  frame True {
                    # "limpa flag"
                    n653 = local write "Flag ativo AH"(FALSE ("Flag ativo AH")) -> ()
                  }
                }
              }
            }
            n654 = call "PROTECAO.vi"("Estado In"=w514) -> ("Estado Out"=w513:i32)  [unwired: 2 in]
            n655 = local write "statAH"(w513) -> ()
            n656 = local read "statCUP"() -> (w520:i32)
            n657 = local read "statDEC"() -> (w521:i32)
            n658 = call "PROTECAO.vi"("Estado In"=w510) -> ("Estado Out"=w496:i32)  [unwired: 2 in]
            n659 = global read "Global_Telescopio.vi" "TargetCUP"() -> (w525:i16)
            n660 = local read "statAH"() -> (w522:i32)
            n661 = global write "Global_Telescopio.vi" "Estado CUP"("statCUP") -> ()
            n662 = global read "Global_Telescopio.vi" "Botão GO = STOP"() -> (w508:bool)
            n663 = local write "statDEC"(w496) -> ()
            n664 = call "Bit Status CUP.vi"("NomeStatus"=w515) -> ("StatBit"=w526:bool)
            n665 = Compound Arithmetic op=ADD(w520, w522, w521) -> (w524:i32)
            n666 = Equal To 0?(x=w524) -> (x = 0?=w523:bool)
            n667 = case shown="2" "statCUP" {
              selector: "statCUP" -> [w545 _ _ _ _ _ _ _]
              tunnel: [w545 w553 w597 1 w607 w628 w638 w656] -> w512
              tunnel: w526 -> [_ w554 _ _ w609 _ w634 _]
              tunnel: w525 -> [_ w549 _ _ _ _ _ _]
              frame 0, Default {
                # "Sem movimento"
                n668 = call "TickTimeout.vi"() -> ("msTick"=→"TimeoutCUP":u32)  [unwired: 2 in, 2 out]
              }
              frame 1 {
                # "20240820"
                # "Envia\nComando"
                n669 = local read "LedPointing"() -> (w550:bool)
                n670 = local read "DOME"() -> (w551:bool)
                n671 = call "Checa destino cupula.vi"("Target"=w549) -> ("moverCup"=w547:bool, "angTarget"=w546:string)  [unwired: 6 in, 1 out]
                n672 = Not(x=w547) -> (.not. x?=w548:bool)
                n673 = case shown="False" w548 {
                  tunnel: w554 -> [w561 w587]
                  tunnel: w549 -> [w560 _]
                  tunnel: [w559 w588] -> w553
                  tunnel: "ChkDomeEnable" -> [w556 w586]
                  tunnel: w551 -> [w558 w585]
                  tunnel: w550 -> [w557 w584]
                  tunnel: w546 -> [w555 _]
                  frame False {
                    # "CUP fora pos."
                    n674 = case shown="False" w561 {
                      tunnel: w560 -> [w569 _]
                      tunnel: [w567 w578] -> w559
                      tunnel: w558 -> [w566 _]
                      tunnel: w557 -> [w564 _]
                      tunnel: w556 -> [w563 _]
                      tunnel: w555 -> [w562 _]
                      frame False {
                        # "CLP Pronto"
                        n675 = Number To Decimal String(number=w569) -> (decimal integer string=w568:string)  [unwired: 1 in]
                        n676 = Select(t=w563, s=w564, f=w566) -> (s? t:f=w565:bool)
                        n677 = case shown="True" w565 {
                          tunnel: [0 2] -> w567
                          tunnel: w568 -> [_ w572]
                          tunnel: w562 -> [_ w571]
                          frame False {
                            # "Cúpula Desabilitada"
                            # "Também não verifica\nTrapeira e Paravento"
                          }
                          frame True {
                            w576 = u16 4 items=["ZERO", "AH", "DEC", "TUBO", "CUP"] ("Controlador")
                            n678 = call "TickTimeout.vi"() -> ("msTick"=w574:u32)  [unwired: 2 in, 2 out]
                            n679 = local write "TargetCup"(w571) -> ()
                            n680 = local write "TimeoutCUP"(w574) -> ()
                            n681 = global write "Global_Telescopio.vi" "T cup"(w574) -> ()
                            n682 = call "Monta Comando.vi"("Set Point"=w572, "Comando"="MOVER", "Dispositivo"="DOMO" ("Comando"), "Controlador"=w576) -> ()  [unwired: 3 in, 3 out]
                          }
                        }
                      }
                      frame True {
                        # "CLP Busy"
                        n683 = local read "TimeoutCUP"() -> (w580:u32)
                        n684 = call "TickTimeout.vi"("msInicial"=w580, "msTimeout"=u32 5000) -> ("Timeout"=w579:bool)  [unwired: 2 out]
                        n685 = case shown="False" w579 {
                          tunnel: [1 3] -> w578
                          frame False {
                          }
                          frame True {
                          }
                        }
                      }
                    }
                  }
                  frame True {
                    # "CUP no destino"
                    n686 = case shown="True" w584 {
                      tunnel: [0 w592] -> w588
                      tunnel: w587 -> [_ _]
                      tunnel: w586 -> [_ w591]
                      tunnel: w585 -> [w589 _]
                      frame False {
                        # "Não está apontando (chave Dome Enable foi ativada)"
                        # "Não verifica\nTrapeira e\nParavento"
                        n687 = local write "Dome on Target"(w589) -> ()
                      }
                      frame True {
                        # "Está apontando"
                        n688 = case shown="True" w591 {
                          tunnel: [0 4] -> w592
                          frame False {
                            # "Não verifica\nTrapeira e\nParavento"
                          }
                          frame True {
                            # "Verifica Trapeira e\nParavento"
                            n689 = call "TickTimeout.vi"() -> ("msTick"=w594:u32)  [unwired: 2 in, 2 out]
                            n690 = local write "TimeoutCUP"(w594) -> ()
                            n691 = global write "Global_Telescopio.vi" "T cup"(w594) -> ()
                          }
                        }
                      }
                    }
                  }
                }
              }
              frame 2 {
                w596 = u16 12 items=["Alarme", "Atencao", "Erro", "Ocupado", "TBD", "LCB", "Trapeira", "Paravento", "DomoRap", "DomoCW", "DomoCCW", "TBD", "Em movimento", "TBD"] ("NomeStatus")
                # "Aqui também caberia um Timeout?"
                # "Aguarda parada motor"
                n692 = call "Bit Status CUP.vi"("NomeStatus"=w596) -> ("StatBit"=w598:bool)
                n693 = case shown="False" w598 {
                  tunnel: [1 2] -> w597
                  frame False {
                    # "Motor parado.\nTestar se chegou\nao destino"
                    n694 = call "TickTimeout.vi"() -> ("msTick"=w599:u32)  [unwired: 2 in, 2 out]
                    n695 = local write "TimeoutCUP"(w599) -> ()
                    n696 = global write "Global_Telescopio.vi" "T cup"(w599) -> ()
                  }
                  frame True {
                    # "Ainda movendo...\nAGUARDAR"
                  }
                }
              }
              frame 3 {
                w605 = u16 4 items=["ZERO", "AH", "DEC", "TUBO", "CUP"] ("Controlador")
                # "Trata Timeout"
                n697 = call "TickTimeout.vi"() -> ("msTick"=w602:u32)  [unwired: 2 in, 2 out]
                n698 = local write "TimeoutCUP"(w602) -> ()
                n699 = global write "Global_Telescopio.vi" "T cup"(w602) -> ()
